vi "Puzzle 3-1.vi"() -> ()   [LabVIEW 2022 SP3]
panel:
  out "sum":i32
  out "Array 3":cluster{i32, i32}[](array[cluster])
  out "Array 2":enum16{"Letter", "Number", "Symbol", "Dot"}[][](array[ring])
  out "Array":string[][](array[string])
  in  "delimited string":string
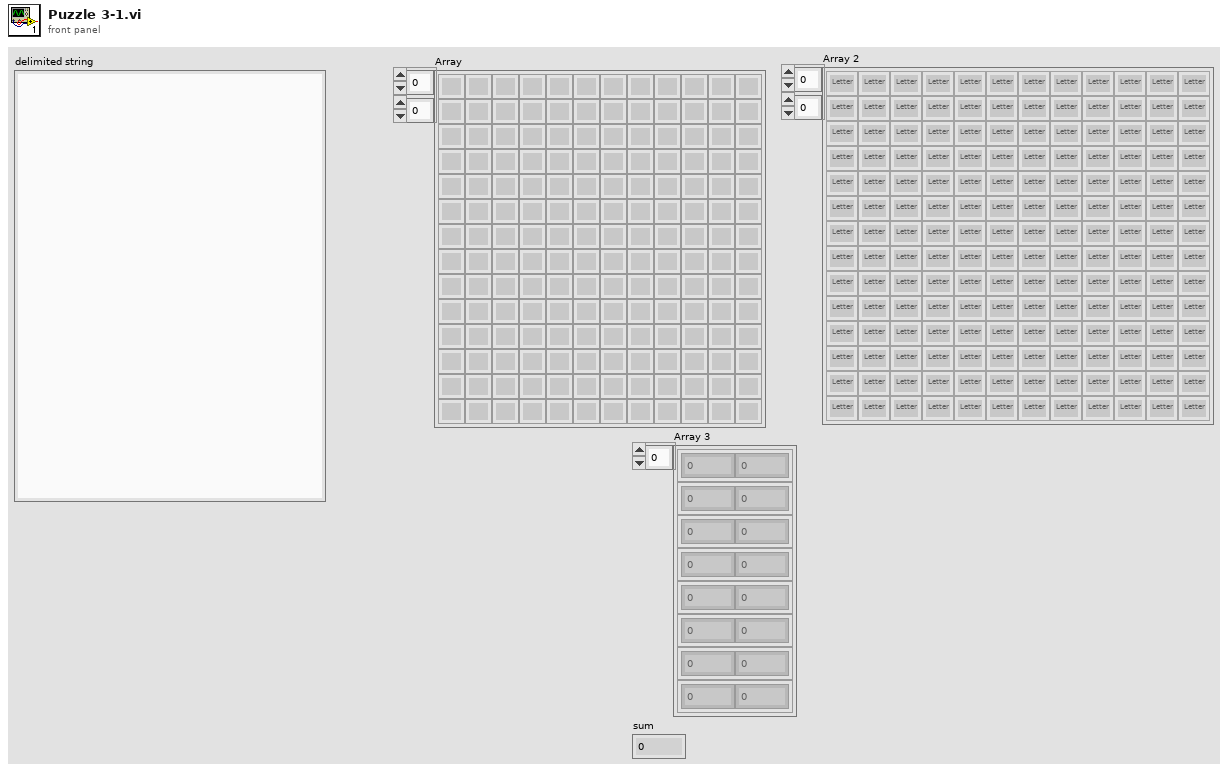
[diagram p1: front panel]
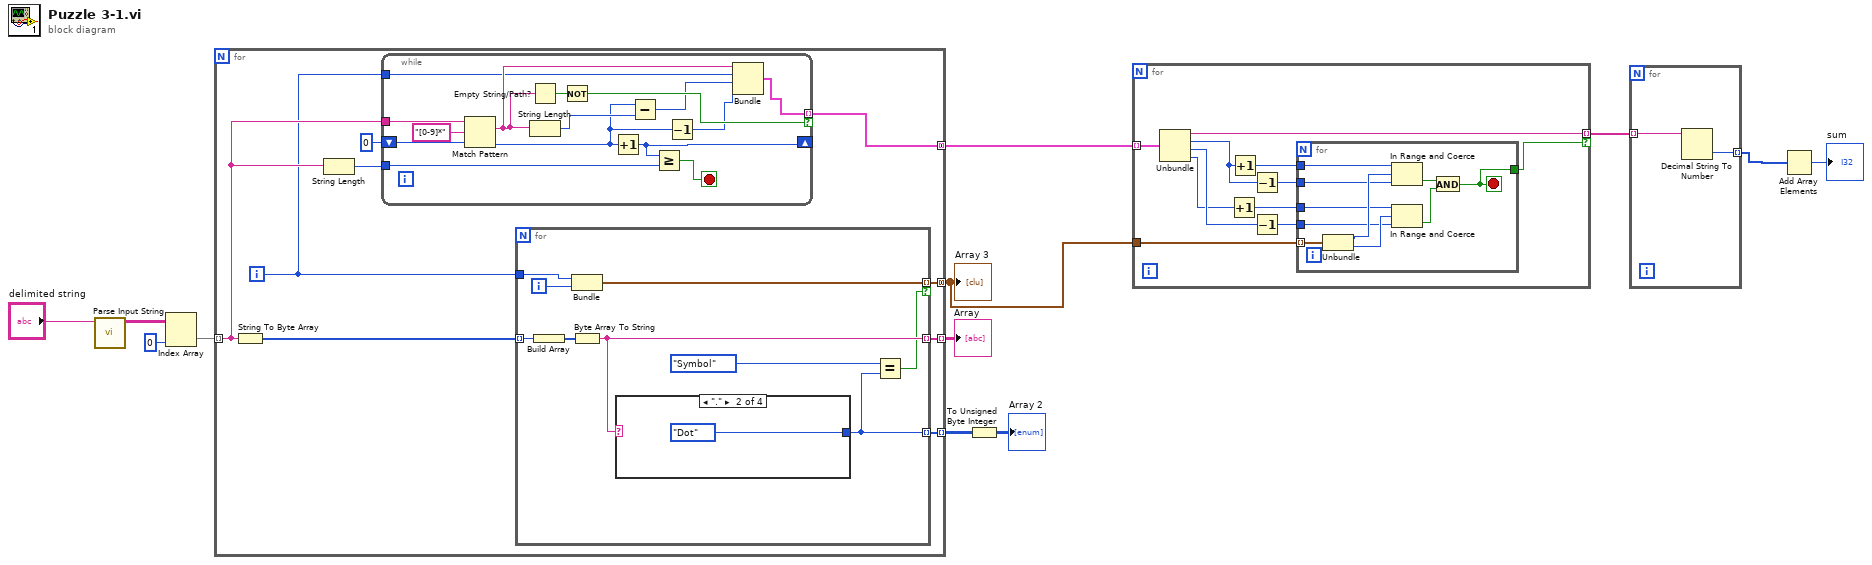
[diagram p0: block diagram]
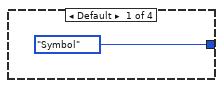
[diagram p2: hidden frame]
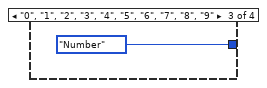
[diagram p3: hidden frame]
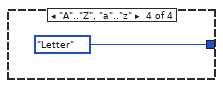
[diagram p4: hidden frame]
diagram:
  n1 = call "Parse Input String.vi"("delimited string"="delimited string") -> ("parsed string"=w11:string[][])  [unwired: 10 in]
  n2 = Index Array(array=w11, index (col)=0 ("disabled index (col)")) -> (element=w9:string[])  [unwired: 1 in]
  n3 = for {
    tunnel: w9 -> [w16] mode=indexing
    tunnel: [w20] -> w8 mode=indexing
    tunnel: [w19] -> w7 mode=indexing
    tunnel: [w18] -> w4 mode=concatenating
    tunnel: [w13] -> w5 mode=concatenating
    i -> [w14]
    n4 = String To Byte Array(string=w16) -> (unsigned byte array=w21:u8[])
    n5 = String Length(string=w16) -> (length=w15:i32)
    n6 = while {
      tunnel: w16 -> [w35]
      tunnel: [w23] -> w13 mode=indexing if=w36
      shift-right: [w29] -> _
      shift-left: 0 -> [w34]
      tunnel: w15 -> [w32]
      tunnel: w14 -> [w22]
      stop <- w30 stop-if-true
      n7 = Match Pattern(string=w35, regular expression="[0-9]*" ("format string"), offset (0)=w34) -> (match substring=w27:string, offset past match=w25:i32)  [unwired: 2 out]
      n8 = Empty String/Path?(string/path=w27) -> (empty?=w31:bool)
      n9 = String Length(string=w27) -> (length=w28:i32)
      n10 = Not(x=w31) -> (.not. x?=w36:bool)
      n11 = Increment(x=w25) -> (x+1=w29:i32)
      n12 = Subtract(x=w25, y=w28) -> (x-y=w26:i32)
      n13 = Greater Or Equal?(x=w29, y=w32) -> (x >= y?=w30:bool)
      n14 = Decrement(x=w25) -> (x-1=w24:i32)
      n15 = Bundle(w27, w22, w26, w24) -> (w23:cluster{string, i32, i32, i32})  [unwired: 1 in]
    }
    n16 = for {
      tunnel: w21 -> [w45] mode=indexing
      tunnel: [w43] -> w20 mode=indexing
      tunnel: [w42] -> w19 mode=indexing
      tunnel: w14 -> [w39]
      tunnel: [w38] -> w18 mode=indexing if=w37
      i -> [w40]
      n17 = Build Array(w45) -> (w44:u8[])
      n18 = Bundle(w39, w40) -> (w38:cluster{i32, i32})  [unwired: 1 in]
      n19 = Byte Array To String(unsigned byte array=w44) -> (string=w43:string)
      n20 = case shown="\".\"" w43 {
        tunnel: [enum16{"Letter", "Number", "Symbol", "Dot"}."Symbol" enum16{"Letter", "Number", "Symbol", "Dot"}."Dot" enum16{"Letter", "Number", "Symbol", "Dot"}."Number" enum16{"Letter", "Number", "Symbol", "Dot"}."Letter"] -> w42
        frame Default {
        }
        frame "." {
        }
        frame "0", "1", "2", "3", "4", "5", "6", "7", "8", "9" {
        }
        frame "A".."Z", "a".."z" {
        }
      }
      n21 = Equal?(x=enum16{"Letter", "Number", "Symbol", "Dot"}."Symbol", y=w42) -> (x = y?=w37:bool)
    }
  }
  "Array" <- w8
  "Array 3" <- w4
  n22 = To Unsigned Byte Integer(number=w7) -> (unsigned 8bit integer=→"Array 2":u8[][])
  n23 = for {
    tunnel: w5 -> [w60] mode=indexing
    tunnel: w4 -> [w56]
    tunnel: [w50] -> w3 mode=indexing if=w51
    n24 = Unbundle(w60) -> (w50:string, w59:i32, w58:i32, w57:i32)
    n25 = Increment(x=w57) -> (x+1=w53:i32)
    n26 = Increment(x=w59) -> (x+1=w54:i32)
    n27 = Decrement(x=w59) -> (x-1=w55:i32)
    n28 = Decrement(x=w58) -> (x-1=w52:i32)
    n29 = for {
      tunnel: w56 -> [w70] mode=indexing
      tunnel: w55 -> [w67]
      tunnel: w54 -> [w66]
      tunnel: w53 -> [w65]
      tunnel: w52 -> [w64]
      tunnel: [w61] -> w51
      stop <- w61 stop-if-true
      n30 = Unbundle(w70) -> (w69:i32, w68:i32)
      n31 = In Range and Coerce(upper limit=w66, x=w69, lower limit=w67) -> (In Range?=w63:bool)  [unwired: 1 out]
      n32 = In Range and Coerce(upper limit=w65, x=w68, lower limit=w64) -> (In Range?=w62:bool)  [unwired: 1 out]
      n33 = And(x=w63, y=w62) -> (x .and. y?=w61:bool)
    }
  }
  n34 = for {
    tunnel: w3 -> [w72] mode=indexing
    tunnel: [w71] -> w2 mode=indexing
    n35 = Decimal String To Number(string=w72) -> (number=w71:i32)  [unwired: 2 in, 1 out]
  }
  n36 = Add Array Elements(numeric array=w2) -> (sum=→"sum":i32)
